vi "fgm_pipeline_mine.vi"(4 "s":bool, 6 "SLMAX":fxp<+/-,18,5>, 7 "StartIndex":u16, 8 "Ns+StartIndex+13":u16, 11 "appended array 2":fxp<+/-,32,3>[](array[numeric])=[0.0, 0.0, 0.0, 0.0, 0.0, 0.0, 0.0, 0.0, 0.0, 0.0, 0.0, 0.0]) -> (2 "appended array":fxp<+/-,32,3>[](array[numeric]))   [LabVIEW 2017]
uses:
  <vilib>/Platform/TimedLoop/XDataNode/timing_clust.ctl
  <vilib>/Platform/TimedLoop/XDataNode/nitl_modes.ctl
  <vilib>/Platform/TimedLoop/XDataNode/wakeup.ctl
  <vilib>/rvi/Emulation/niFpgaSctlEmulationGetInTimedLoop.vi
  <vilib>/rvi/Emulation/niFpgaEmulationReportErrorSimple.vi
  <vilib>/rvi/Emulation/niFpgaGetClockAttributes.vi
  <vilib>/rvi/Emulation/niFpgaCriticalErrorInLSC.vi
  <vilib>/Platform/TimedLoop/XDataNode/XDataNode.xnode
  <vilib>/Platform/TimedLoop/XDataNode/XDNodeRunTimeDep.lvlib
panel:
  out "Numeric":i32
  in  "Ns":i16
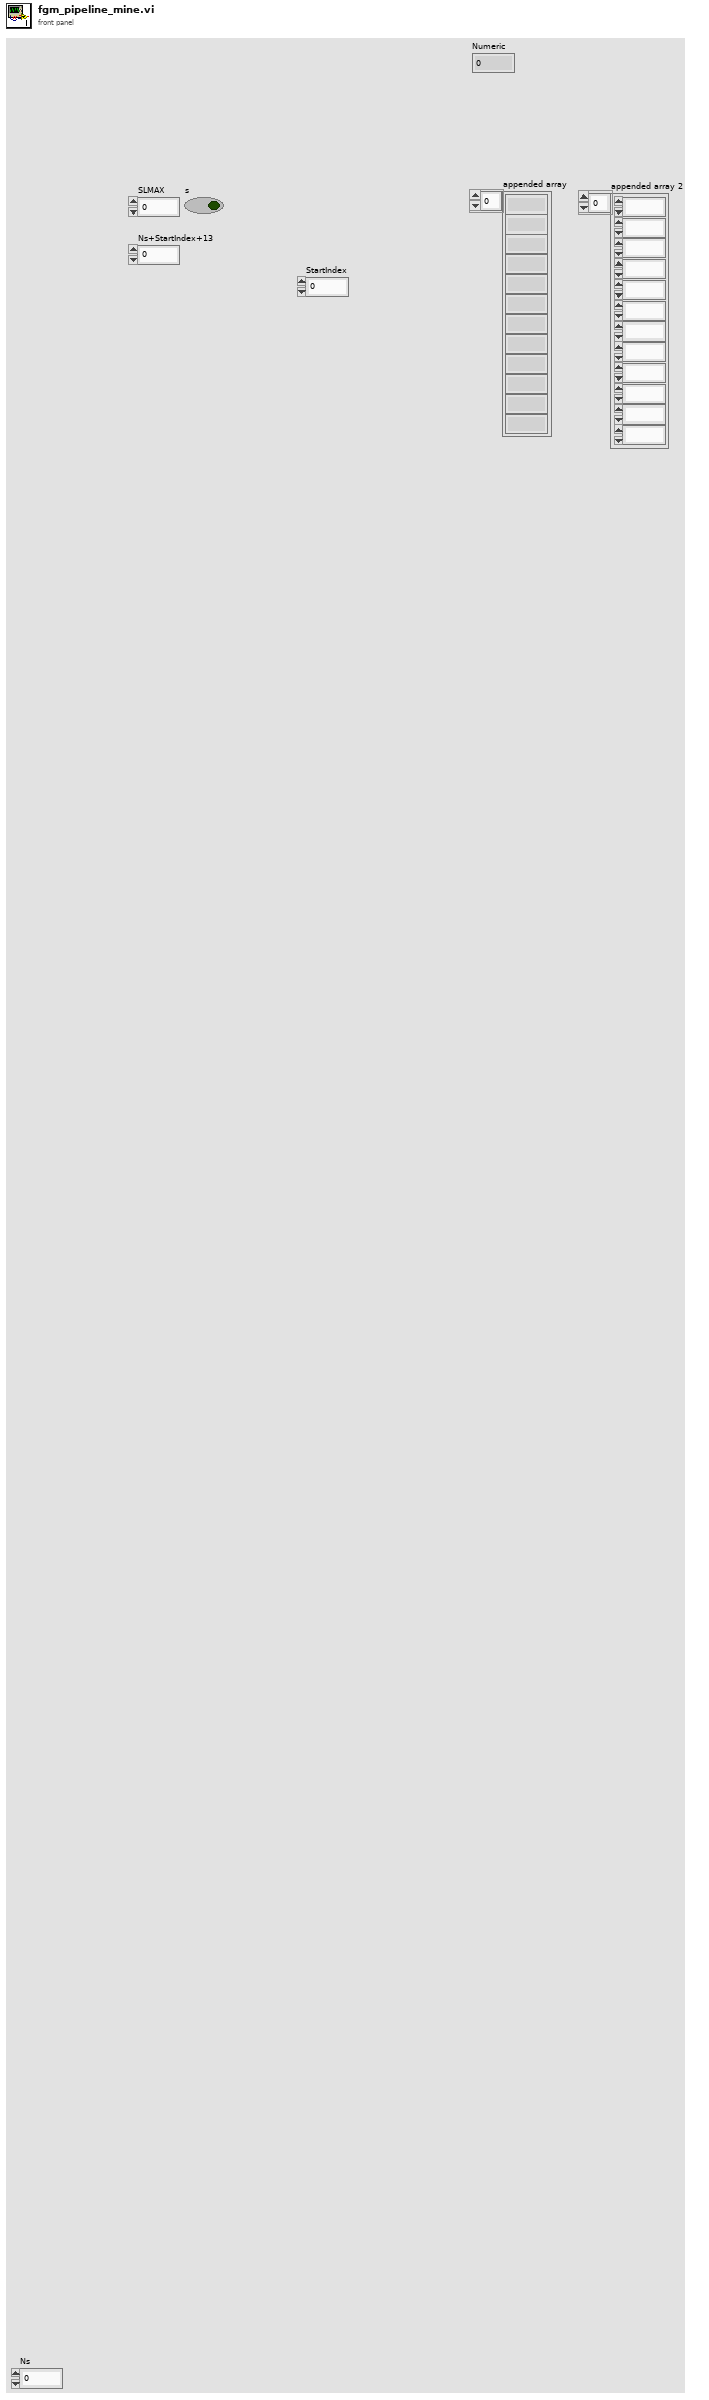
[diagram p1: front panel]
types:
  T1 = typedef "XDNodeRunTimeDep.lvlib/timing_clust.ctl" = cluster{"Expected End [f-1]":u64, "Actual End [f-1]":u64, "Finished Late? [f-1]":bool, "Expected End [i-1]":u64, "Actual End [i-1]":u64, "Finished Late? [i-1]":bool, "Expected Start [i]":u64, "Actual Start [i]":u64, "Expected Start [f]":u64, "Actual Start [f]":u64, "Source Name":string, "Structure Name":string, "Period":i64, "Deadline":i64, "Offset":i64, "Start":i64, "Priority":i32, "Timeout":i32, "Mode":T2, "Wakeup Reason":T3, "Error":errorcluster, "Source Type":string, "Secondary Source Type":string, "Global End Time":u64, "Global Start Time":u64, "Frame Duration":u64, "Iteration Duration":u64, "Assigned CPU":i32, "I/O Scan Engine Mode":u32}
  T2 = typedef "XDNodeRunTimeDep.lvlib/nitl_modes.ctl" = enum32{"No Change", "Process missed periods, maintain original phase", "Discard missed periods, maintain original phase", "Process missed periods, ignore original phase", "Discard missed periods, ignore original phase"}
  T3 = typedef "XDNodeRunTimeDep.lvlib/wakeup.ctl" = enum32{"Normal", "Aborted", "Asynchronous wakeup", "Timing source error", "Timed loop error", "Timeout"}
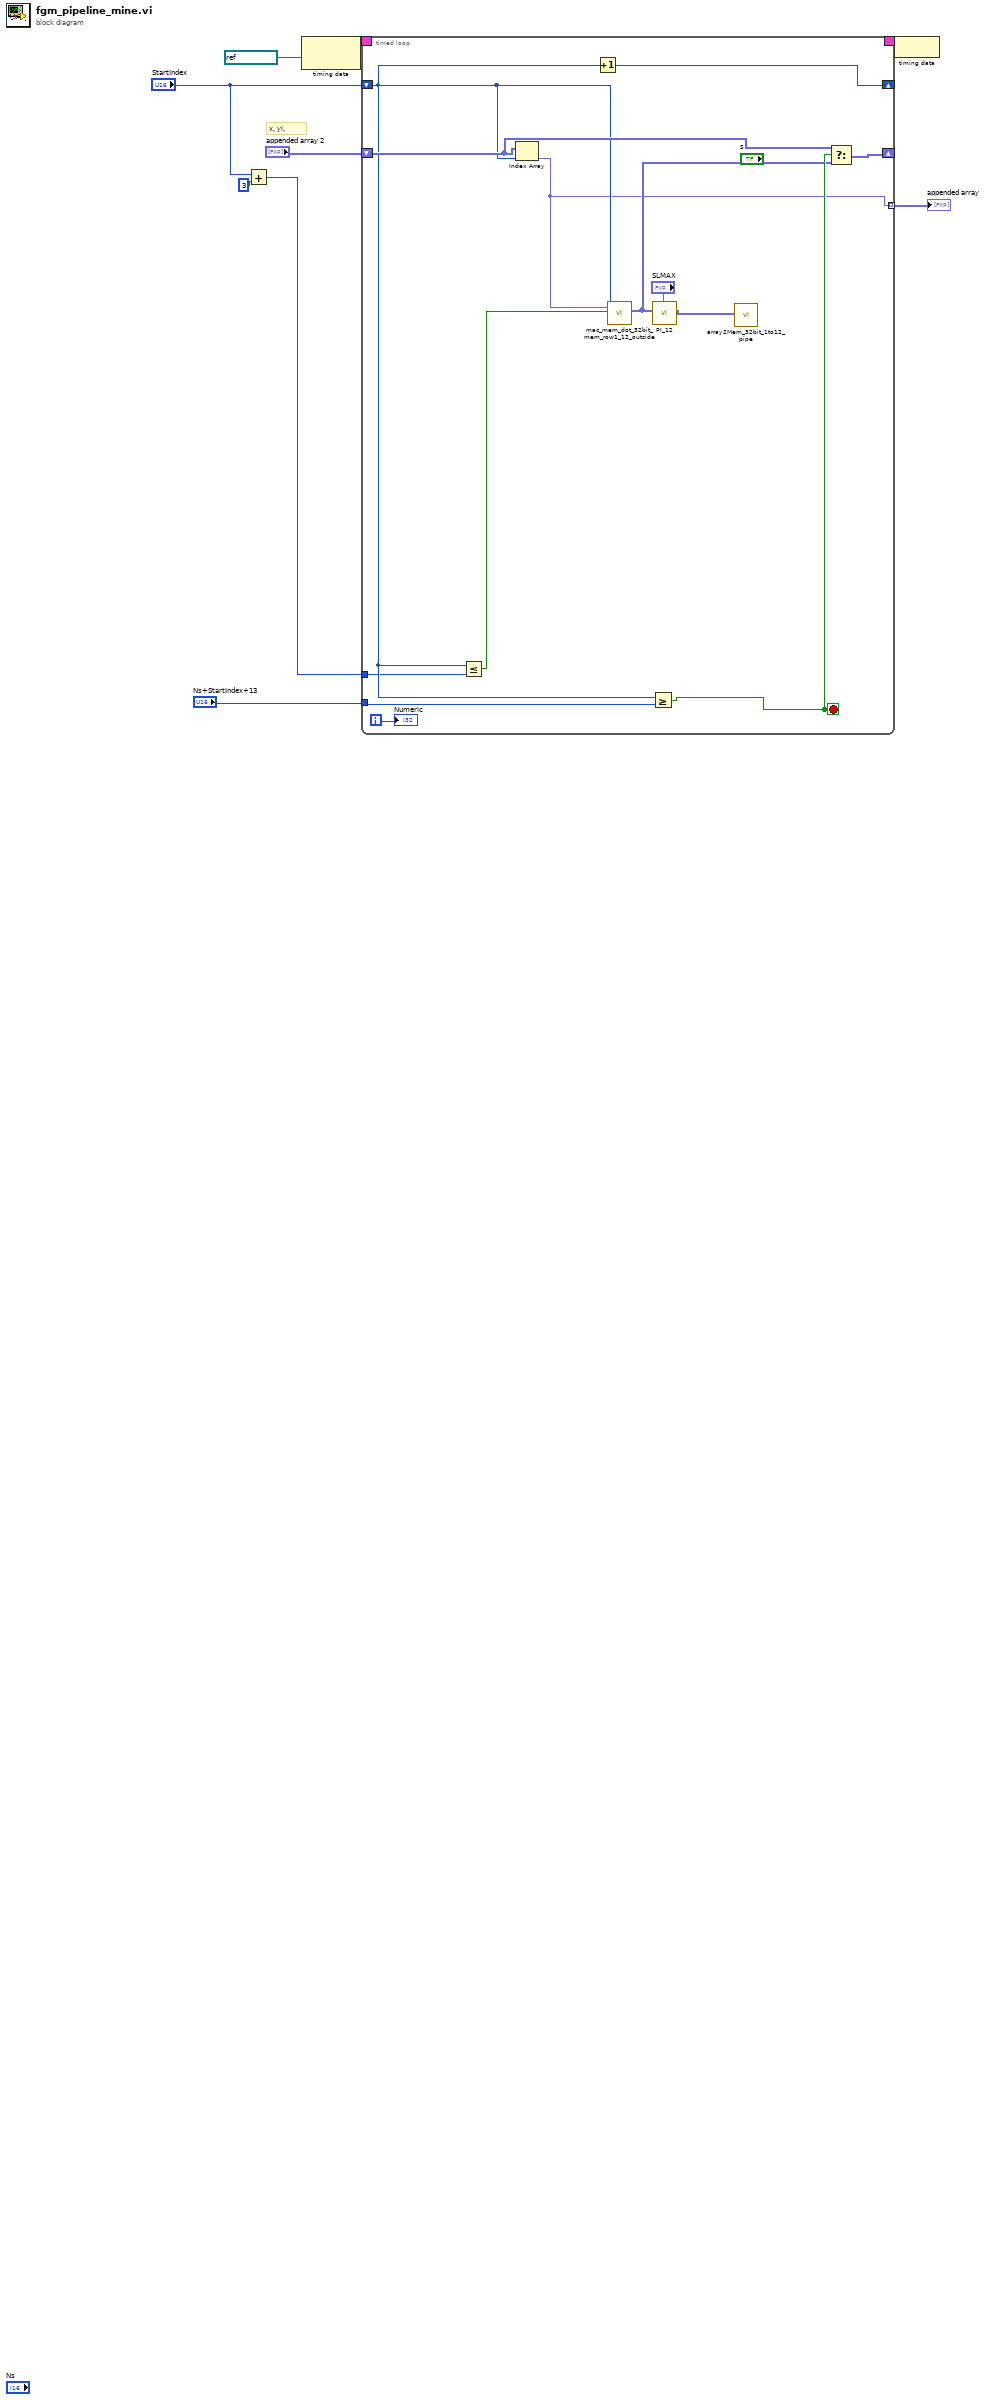
[diagram p0: block diagram]
diagram:
  # "x, yi,"
  n1 = Add(x="StartIndex", y=i16 3) -> (x+y=w4:u16)
  n2 = node-c288(refnum<k21> "100MHz" ("Source Name")) -> (w9:T1)
  n3 = timed-loop {
    timing: w9 -> [_]
    timing-out: [_] -> w8
    tunnel: "Ns+StartIndex+13" -> [w22]
    shift-right: [w21] -> _
    shift-left: "StartIndex" -> [w13]
    tunnel: w4 -> [w12]
    shift-right: [w17] -> _
    shift-left: "appended array 2" -> [w18]
    tunnel: [w10] -> w2 mode=indexing
    i -> [w11]
    stop <- w16 stop-if-true
    n4 = Less Or Equal?(x=w13, y=w12) -> (x <= y?=w14:bool)
    n5 = Index Array(array=w18, index=w13) -> (element=w10:fxp<+/-,32,3>)
    n6 = Increment(x=w13) -> (x+1=w21:u16)
    n7 = call "mac_mem_dot_32bit_mem_row1_12_outside.vi"("StartIndex"=w13, "x_i"=w10, "Boolean"=w14) -> ("appended array"=w15:fxp<+/-,32,3>[])  [unwired: 16 in]
    n8 = Greater Or Equal?(x=w13, y=w22) -> (x >= y?=w16:bool)
    n9 = call "PI_12.vi"("SLMAX"="SLMAX", "array in"=w15) -> ("appended array"=w19:fxp<+/-,32,3>[])  [unwired: 9 in]
    n10 = call "array2Mem_32bit_1to12_pipe.vi"("array in"=w19) -> ()  [unwired: 11 in]
    n11 = Select(t=w18, s=w16, f=w15) -> (s? t:f=w17:fxp<+/-,32,3>[])
    "Numeric" <- w11
  }
  "appended array" <- w2
  n12 = node-c288(w8) -> ()
